vi "GetPointQuadrant.vi"(5 "Point":cluster{"X":sgl, "Y":sgl, "Z":sgl}) -> (2 "Quadrant":i32)   [LabVIEW 2014]
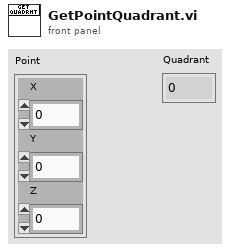
[diagram p1: front panel]
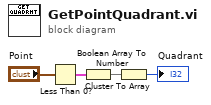
[diagram p0: block diagram]
diagram:
  n1 = Less Than 0?(x="Point") -> (x < 0?=w3:cluster{"X":bool, "Y":bool, "Z":bool})
  n2 = Cluster To Array(cluster=w3) -> (array=w2:bool[])
  n3 = Boolean Array To Number(Boolean array=w2) -> (number=→"Quadrant":u32)
